vi "volinfo.vi"(7 "File Sys Name Size":u32=100, 8 "Volume Name Size":u32=100, 9 "Root Path Name":string="C:\\") -> (0 "File System Flags":u32, 1 "Max Component Length":u32, 2 "Volume Serial Number":string, 3 "Volume Name":string, 4 "File System Name":string)   [LabVIEW 2014]
doc: "The Get Volume Information function returns information about a file system and volume whose root directory is specified."
uses:
  KERNEL32.DLL
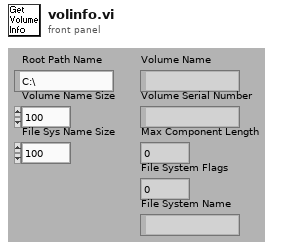
[diagram p1: front panel]
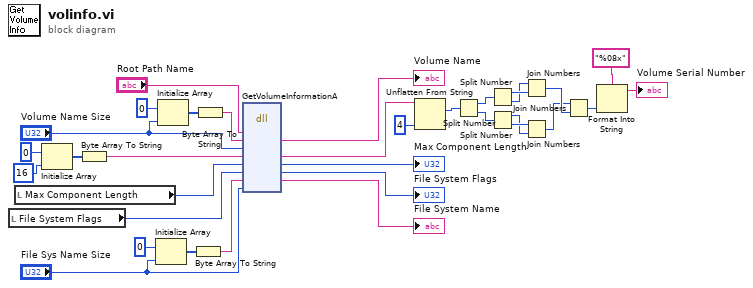
[diagram p0: block diagram]
diagram:
  n1 = local read "File System Flags"() -> (w20:u32)
  n2 = local read "Max Component Length"() -> (w21:u32)
  n3 = Initialize Array(u8 0, 16 ("dimension size")) -> (w2:u8[])
  n4 = Byte Array To String(unsigned byte array=w2) -> (string=w1:string)
  n5 = Initialize Array(u8 0, "File Sys Name Size") -> (w25:u8[])
  n6 = Initialize Array(u8 0, "Volume Name Size") -> (w27:u8[])
  n7 = Byte Array To String(unsigned byte array=w25) -> (string=w23:string)
  n8 = Byte Array To String(unsigned byte array=w27) -> (string=w26:string)
  n9 = dll-call lib="KERNEL32.DLL" fn="GetVolumeInformationA"("lpRootPathName"="Root Path Name", "lpVolumeNameBuffer"=w26, "nVolumeNameSize"="Volume Name Size", "lpVolumeSerialNumber"=w1, "lpMaximumComponentLength"=w21, "lpFileSystemFlags"=w20, "lpFileSystemNameBuffer"=w23, "nFileSystemNameSize"="File Sys Name Size") -> ("lpVolumeNameBuffer"=→"Volume Name":string, "lpVolumeSerialNumber"=w18:string, "lpMaximumComponentLength"=→"Max Component Length":u32, "lpFileSystemFlags"=→"File System Flags":u32, "lpFileSystemNameBuffer"=→"File System Name":string)  [unwired: 7 in, 2 out]
  n10 = Unflatten From String(type=u32 4 ("length (rest)"), binary string=w18) -> (value=w16:u32)  [unwired: 3 in, 2 out]
  n11 = Split Number(x=w16) -> (hi(x)=w14:u16, lo(x)=w13:u16)
  n12 = Split Number(x=w14) -> (hi(x)=w7:u8, lo(x)=w6:u8)
  n13 = Split Number(x=w13) -> (hi(x)=w8:u8, lo(x)=w9:u8)
  n14 = Join Numbers(hi=w6, lo=w7) -> ((hi.lo)=w12:u16)
  n15 = Join Numbers(hi=w9, lo=w8) -> ((hi.lo)=w11:u16)
  n16 = Join Numbers(hi=w11, lo=w12) -> ((hi.lo)=w10:u32)
  n17 = Format Into String(format string="%08x" ("Format String"), w10) -> (resulting string=→"Volume Serial Number":string)  [unwired: 2 in, 1 out]
